vi "GFITS_WriteHeaders_1ext.vi"(0 "ref":u64, 1 "extension":i32, 2 "Database RefNum in":T1, 7 "Keywords":string[][](array[string]), 9 "numer of keywords":i32, 11 "error in (no error)":errorcluster, 12 "expID in":string) -> (6 "ref out":u64, 10 "expID":string, 15 "error out":errorcluster)   [LabVIEW 2016]
uses:
  GFITS_datatypesctl.ctl
  DBSHAND/private/vis/DatabaseHand_RefNum.ctl
  DBSHAND/private/vis/DatabaseHand_Element_Get(bool).vi
panel:
  in  "Types":T2={"TBIT"=1, "TBYTE"=11, "TSTRING"=16, "TSHORT"=21, "TLONG"=41, "TFLOAT"=42, "TDOUBLE"=82, "TCOMPLEX"=83, "TDBLCOMPLEX"=163, "TUINT"=30, "TUSHORT"=20, "TULONG"=40, "TINT"=31, "TSBYTE"=12, "TLONGLONG"=81, "TLOGICAL"=14}
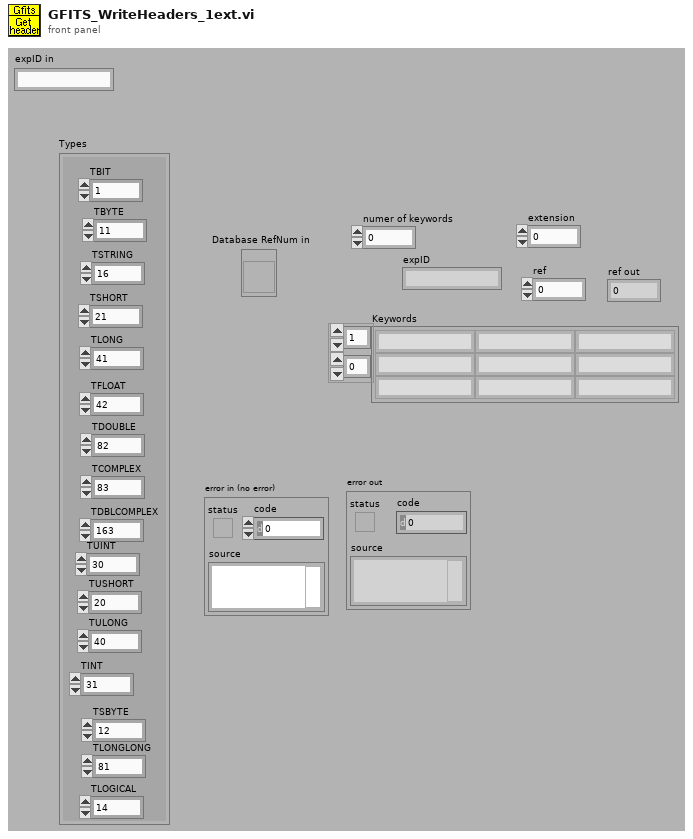
[diagram p1: front panel]
types:
  T1 = typedef "DatabaseHand_RefNum.ctl" = refnum<vi>
  T2 = typedef "GFITS_datatypesctl.ctl" = cluster{"TBIT":i32, "TBYTE":i32, "TSTRING":i32, "TSHORT":i32, "TLONG":i32, "TFLOAT":i32, "TDOUBLE":i32, "TCOMPLEX":i32, "TDBLCOMPLEX":i32, "TUINT":i32, "TUSHORT":i32, "TULONG":i32, "TINT":i32, "TSBYTE":i32, "TLONGLONG":i32, "TLOGICAL":i32}
  T3 = enum16{"clear all", "add extension", "add keyword", "get", "clear extension", "done"}
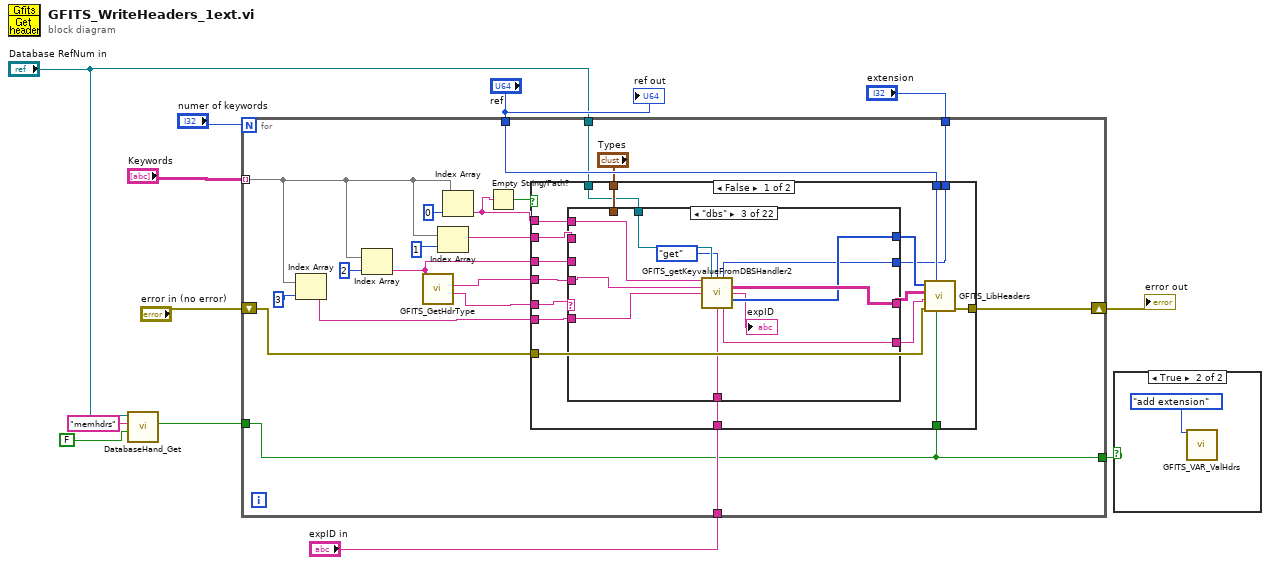
[diagram p0: block diagram]
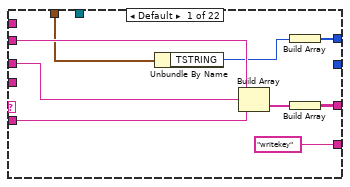
[diagram p3: hidden frame]
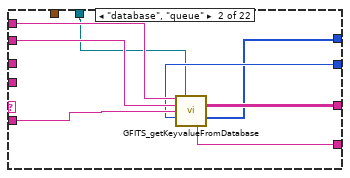
[diagram p4: hidden frame]
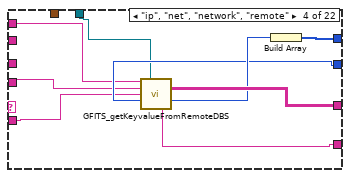
[diagram p5: hidden frame]
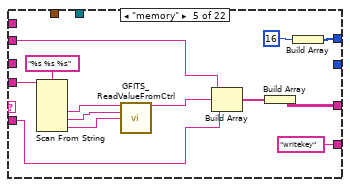
[diagram p6: hidden frame]
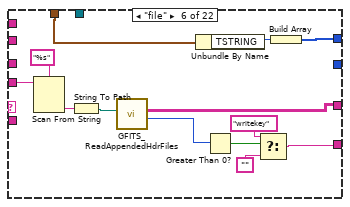
[diagram p7: hidden frame]
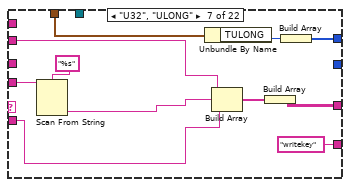
[diagram p8: hidden frame]
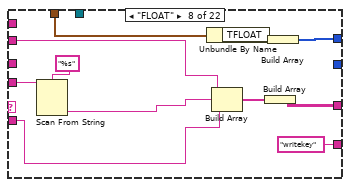
[diagram p9: hidden frame]
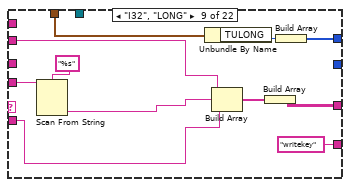
[diagram p10: hidden frame]
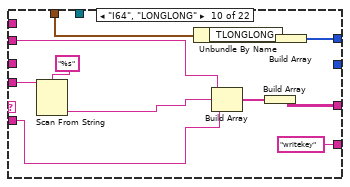
[diagram p11: hidden frame]
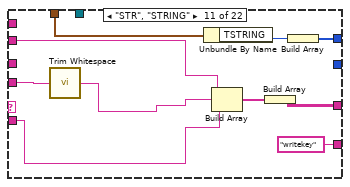
[diagram p12: hidden frame]
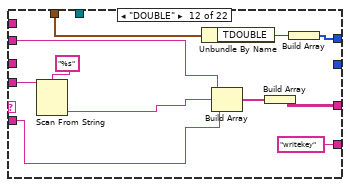
[diagram p13: hidden frame]
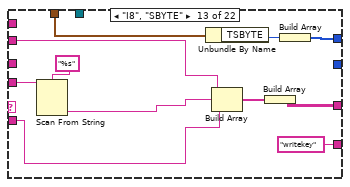
[diagram p14: hidden frame]
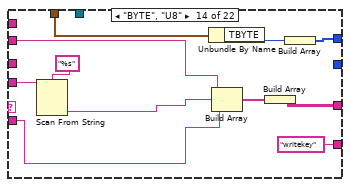
[diagram p15: hidden frame]
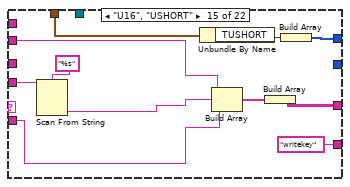
[diagram p16: hidden frame]
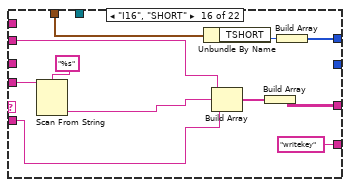
[diagram p17: hidden frame]
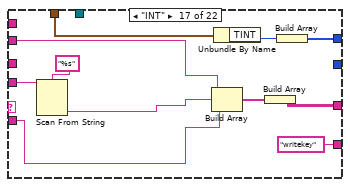
[diagram p18: hidden frame]
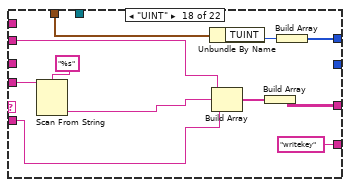
[diagram p19: hidden frame]
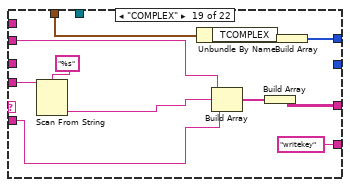
[diagram p20: hidden frame]
diagram:
  n1 = call-poly "DatabaseHand_Get.vi"("default value"=FALSE, "name"="memhdrs", "Database RefNum in"="Database RefNum in") -> ("value"=w2:bool)  [unwired: 2 in, 6 out]
  n2 = for {
    N: "numer of keywords" -> [_]
    tunnel: "Keywords" -> [w26] mode=indexing
    tunnel: "ref" -> [w27]
    tunnel: "extension" -> [w21]
    shift-right: [w16] -> w9
    shift-left: "error in (no error)" -> [w20]
    tunnel: "Database RefNum in" -> [w19]
    tunnel: "expID in" -> [w14]
    tunnel: w2 -> [w13]
    tunnel: [w13] -> w1
    n3 = Index Array(array=w26, index=3 ("Array Index")) -> (element=w28:string)
    n4 = Index Array(array=w26, index=2 ("Array Index")) -> (element=w15:string)
    n5 = call "GFITS_GetHdrType.vi"("keyval"=w15) -> ("type"=w18:string, "keyval out"=w17:string)  [unwired: 9 out]
    n6 = Index Array(array=w26, index=1 ("Array Index")) -> (element=w29:string)
    n7 = Index Array(array=w26, index=0 ("Index")) -> (element=w24:string)
    n8 = Empty String/Path?(string/path=w24) -> (empty?=w23:bool)
    n9 = case shown="False" w23 {
      tunnel: w29 -> [w47 _]
      tunnel: w28 -> [w44 _]
      tunnel: w18 -> [w45 _]
      tunnel: w17 -> [w46 _]
      tunnel: w27 -> [w49 _]
      tunnel: w24 -> [w48 _]
      tunnel: "Types" -> [w41 _]
      tunnel: w21 -> [w35 _]
      tunnel: [w40 w287] -> w16
      tunnel: w20 -> [w39 w287]
      tunnel: w19 -> [w36 _]
      tunnel: w15 -> [w38 _]
      tunnel: w14 -> [w37 _]
      tunnel: w13 -> [w33 _]
      frame False {
        n10 = case shown="\"dbs\"" w45 {
          tunnel: w44 -> [w56 w65 w74 w80 w91 _ w119 w130 w141 w152 w164 w173 w184 w195 w206 w217 w228 w239 w250 w261 w272 w284]
          tunnel: ["writekey" w66 w71 w86 "writekey" ("function to use") w101 "writekey" ("function to use") "writekey" ("function to use") "writekey" ("function to use") "writekey" ("function to use") "writekey" ("function to use") "writekey" ("function to use") "writekey" ("function to use") "writekey" ("function to use") "writekey" ("function to use") "writekey" ("function to use") "writekey" ("function to use") "writekey" ("function to use") "writekey" ("function to use") "writekey" ("function to use") "writekey" ("function to use") "writekey" ("function to use")] -> w42
          tunnel: [w53 w59 w72 w78 w87 w100 w113 w124 w135 w146 w157 w167 w178 w189 w200 w211 w222 w233 w244 w255 w266 w281] -> w43
          tunnel: w47 -> [w57 w62 _ _ w92 _ w120 w131 w142 w153 w165 w174 w185 w196 w207 w218 w229 w240 w251 w262 w273 w285]
          tunnel: w46 -> [_ _ w75 w81 w99 w110 w123 w134 w145 w156 w159 w177 w188 w199 w210 w221 w232 w243 w254 w265 w276 w280]
          tunnel: [w54 w64 w73 w85 w88 w104 w117 w128 w139 w150 w162 w171 w182 w193 w204 w215 w226 w237 w248 w259 w270 w282] -> w34
          tunnel: w48 -> [_ w63 w76 w82 _ _ _ _ _ _ _ _ _ _ _ _ _ _ _ _ _ _]
          tunnel: w41 -> [w52 _ _ _ _ w112 w115 w126 w137 w148 w161 w169 w180 w191 w202 w213 w224 w235 w246 w257 w268 _]
          tunnel: w35 -> [_ w61 w68 w83 _ _ _ _ _ _ _ _ _ _ _ _ _ _ _ _ _ _]
          tunnel: w36 -> [_ w60 w77 w79 _ _ _ _ _ _ _ _ _ _ _ _ _ _ _ _ _ w279]
          tunnel: w38 -> [w50 _ _ _ _ _ _ _ _ _ _ _ _ _ _ _ _ _ _ _ _ _]
          tunnel: w37 -> [_ _ w67 _ _ _ _ _ _ _ _ _ _ _ _ _ _ _ _ _ _ _]
          frame Default {
            n11 = Unbundle By Name(w52) -> ("TSTRING"=w51:i32)
            n12 = Build Array(w57, w50, w56) -> (w55:string[])
            n13 = Build Array(w51) -> (w53:i32[])
            n14 = Build Array(w55) -> (w54:string[][])
          }
          frame "database", "queue" {
            n15 = call "GFITS_getKeyvalueFromDatabase.vi"("key name in header"=w63, "Database RefNum in"=w60, "Keyname"=w62, "comment"=w65, "extension"=w61) -> ("table out"=w64:string[][], "datatype"=w59:u16[], "function to use"=w66:string)  [unwired: 1 in, 7 out]
          }
          frame "dbs" {
            n16 = call "GFITS_getKeyvalueFromDBSHandler2.vi"("key name in header"=w76, "Database RefNum in"=w77, "action"=enum16{"get", "clear"}."get", "extension"=w68, "varname"=w75, "comment"=w74, "expID in"=w67) -> ("table out"=w73:string[][], "expID"=→"expID":string, "datatype"=w72:u16[], "function to use"=w71:string)  [unwired: 3 in, 2 out]
          }
          frame "ip", "net", "network", "remote" {
            n17 = call "GFITS_getKeyvalueFromRemoteDBS.vi"("key name in header"=w82, "Database RefNum in"=w79, "varname"=w81, "comment"=w80, "extension"=w83) -> ("table out"=w85:string[][], "datatype"=w84:u16, "function to use"=w86:string)  [unwired: 1 in, 7 out]
            n18 = Build Array(w84) -> (w78:u16[])
          }
          frame "memory" {
            n19 = Scan From String(format string="%s %s %s" ("Format String"), input string=w99) -> (output 1=w97:string, output 2=w96:string, output 3=w95:string)  [unwired: 2 in, 6 out]
            n20 = call "GFITS_ReadValueFromCtrl.vi"("Vi name"=w97, "Control Name"=w96, "Type"=w95) -> ("Value"=w90:string)  [unwired: 1 in, 11 out]
            n21 = Build Array(w92, w90, w91) -> (w89:string[])
            n22 = Build Array(w89) -> (w88:string[][])
            n23 = Build Array(16 ("datatype")) -> (w87:i32[])
          }
          frame "file" {
            n24 = Scan From String(format string="%s", input string=w110) -> (output 1=w108:string)  [unwired: 2 in, 4 out]
            n25 = String To Path(string=w108) -> (path=w107:path)
            n26 = call "GFITS_ReadAppendedHdrFiles.vi"("Path"=w107) -> ("keywords found"=w106:i32, "Array"=w104:string[][])  [unwired: 1 in, 8 out]
            n27 = Unbundle By Name(w112) -> ("TSTRING"=w111:i32)
            n28 = Greater Than 0?(x=w106) -> (x > 0?=w105:bool)
            n29 = Select(t="writekey" ("function to use"), s=w105, f="") -> (s? t:f=w101:string)
            n30 = Build Array(w111) -> (w100:i32[])
          }
          frame "U32", "ULONG" {
            n31 = Scan From String(format string="%s" ("Format String"), input string=w123) -> (output 1=w116:string)  [unwired: 2 in, 4 out]
            n32 = Unbundle By Name(w115) -> ("TULONG"=w114:i32)
            n33 = Build Array(w120, w116, w119) -> (w118:string[])
            n34 = Build Array(w118) -> (w117:string[][])
            n35 = Build Array(w114) -> (w113:i32[])
          }
          frame "FLOAT" {
            n36 = Scan From String(format string="%s" ("Format String"), input string=w134) -> (output 1=w127:string)  [unwired: 2 in, 4 out]
            n37 = Unbundle By Name(w126) -> ("TFLOAT"=w125:i32)
            n38 = Build Array(w131, w127, w130) -> (w129:string[])
            n39 = Build Array(w129) -> (w128:string[][])
            n40 = Build Array(w125) -> (w124:i32[])
          }
          frame "I32", "LONG" {
            n41 = Scan From String(format string="%s" ("Format String"), input string=w145) -> (output 1=w138:string)  [unwired: 2 in, 4 out]
            n42 = Unbundle By Name(w137) -> ("TULONG"=w136:i32)
            n43 = Build Array(w142, w138, w141) -> (w140:string[])
            n44 = Build Array(w140) -> (w139:string[][])
            n45 = Build Array(w136) -> (w135:i32[])
          }
          frame "I64", "LONGLONG" {
            n46 = Scan From String(format string="%s" ("Format String"), input string=w156) -> (output 1=w149:string)  [unwired: 2 in, 4 out]
            n47 = Unbundle By Name(w148) -> ("TLONGLONG"=w147:i32)
            n48 = Build Array(w153, w149, w152) -> (w151:string[])
            n49 = Build Array(w151) -> (w150:string[][])
            n50 = Build Array(w147) -> (w146:i32[])
          }
          frame "STR", "STRING" {
            n51 = call <vilib>:"Trim Whitespace.vi"("string"=w159) -> ("trimmed string"=w158:string)  [unwired: 1 in]
            n52 = Unbundle By Name(w161) -> ("TSTRING"=w160:i32)
            n53 = Build Array(w165, w158, w164) -> (w163:string[])
            n54 = Build Array(w163) -> (w162:string[][])
            n55 = Build Array(w160) -> (w157:i32[])
          }
          frame "DOUBLE" {
            n56 = Scan From String(format string="%s" ("Format String"), input string=w177) -> (output 1=w170:string)  [unwired: 2 in, 4 out]
            n57 = Unbundle By Name(w169) -> ("TDOUBLE"=w168:i32)
            n58 = Build Array(w174, w170, w173) -> (w172:string[])
            n59 = Build Array(w172) -> (w171:string[][])
            n60 = Build Array(w168) -> (w167:i32[])
          }
          frame "I8", "SBYTE" {
            n61 = Scan From String(format string="%s" ("Format String"), input string=w188) -> (output 1=w181:string)  [unwired: 2 in, 4 out]
            n62 = Unbundle By Name(w180) -> ("TSBYTE"=w179:i32)
            n63 = Build Array(w185, w181, w184) -> (w183:string[])
            n64 = Build Array(w183) -> (w182:string[][])
            n65 = Build Array(w179) -> (w178:i32[])
          }
          frame "BYTE", "U8" {
            n66 = Scan From String(format string="%s" ("Format String"), input string=w199) -> (output 1=w192:string)  [unwired: 2 in, 4 out]
            n67 = Unbundle By Name(w191) -> ("TBYTE"=w190:i32)
            n68 = Build Array(w196, w192, w195) -> (w194:string[])
            n69 = Build Array(w194) -> (w193:string[][])
            n70 = Build Array(w190) -> (w189:i32[])
          }
          frame "U16", "USHORT" {
            n71 = Scan From String(format string="%s" ("Format String"), input string=w210) -> (output 1=w203:string)  [unwired: 2 in, 4 out]
            n72 = Unbundle By Name(w202) -> ("TUSHORT"=w201:i32)
            n73 = Build Array(w207, w203, w206) -> (w205:string[])
            n74 = Build Array(w205) -> (w204:string[][])
            n75 = Build Array(w201) -> (w200:i32[])
          }
          frame "I16", "SHORT" {
            n76 = Scan From String(format string="%s" ("Format String"), input string=w221) -> (output 1=w214:string)  [unwired: 2 in, 4 out]
            n77 = Unbundle By Name(w213) -> ("TSHORT"=w212:i32)
            n78 = Build Array(w218, w214, w217) -> (w216:string[])
            n79 = Build Array(w216) -> (w215:string[][])
            n80 = Build Array(w212) -> (w211:i32[])
          }
          frame "INT" {
            n81 = Scan From String(format string="%s" ("Format String"), input string=w232) -> (output 1=w225:string)  [unwired: 2 in, 4 out]
            n82 = Build Array(w229, w225, w228) -> (w227:string[])
            n83 = Unbundle By Name(w224) -> ("TINT"=w223:i32)
            n84 = Build Array(w227) -> (w226:string[][])
            n85 = Build Array(w223) -> (w222:i32[])
          }
          frame "UINT" {
            n86 = Scan From String(format string="%s" ("Format String"), input string=w243) -> (output 1=w236:string)  [unwired: 2 in, 4 out]
            n87 = Unbundle By Name(w235) -> ("TUINT"=w234:i32)
            n88 = Build Array(w240, w236, w239) -> (w238:string[])
            n89 = Build Array(w238) -> (w237:string[][])
            n90 = Build Array(w234) -> (w233:i32[])
          }
          frame "COMPLEX" {
            n91 = Scan From String(format string="%s" ("Format String"), input string=w254) -> (output 1=w247:string)  [unwired: 2 in, 4 out]
            n92 = Unbundle By Name(w246) -> ("TCOMPLEX"=w245:i32)
            n93 = Build Array(w251, w247, w250) -> (w249:string[])
            n94 = Build Array(w249) -> (w248:string[][])
            n95 = Build Array(w245) -> (w244:i32[])
          }
          frame "DBLCOMPLEX" {
            n96 = Scan From String(format string="%s" ("Format String"), input string=w265) -> (output 1=w258:string)  [unwired: 2 in, 4 out]
            n97 = Unbundle By Name(w257) -> ("TDBLCOMPLEX"=w256:i32)
            n98 = Build Array(w262, w258, w261) -> (w260:string[])
            n99 = Build Array(w260) -> (w259:string[][])
            n100 = Build Array(w256) -> (w255:i32[])
          }
          frame "BIT", "BOOL" {
            n101 = Scan From String(format string="%s" ("Format String"), input string=w276) -> (output 1=w269:string)  [unwired: 2 in, 4 out]
            n102 = Build Array(w273, w269, w272) -> (w271:string[])
            n103 = Unbundle By Name(w268) -> ("TBIT"=w267:i32)
            n104 = Build Array(w271) -> (w270:string[][])
            n105 = Build Array(w267) -> (w266:i32[])
          }
          frame "evaluate", "expression", "operate" {
            n106 = call "GFITS_header_operate.vi"("expression"=w280, "Database RefNum in"=w279) -> ("value"=w277:string, "numeric data type"=w278:i32)  [unwired: 8 out]
            n107 = Build Array(w285, w277, w284) -> (w283:string[])
            n108 = Build Array(w283) -> (w282:string[][])
            n109 = Build Array(w278) -> (w281:i32[])
          }
        }
        n110 = call "GFITS_LibHeaders.vi"("memheaders"=w33, "file ref"=w49, "error in (no error)"=w39, "funtion name"=w42, "Table In"=w34, "data type"=w43) -> ("error out"=w40:errorcluster)  [unwired: 5 out]
      }
      frame True {
      }
    }
  }
  "error out" <- w9
  n111 = case shown="True" w1 {
    frame False {
    }
    frame True {
      n112 = call "GFITS_VAR_ValHdrs.vi"("action"=T3."add extension") -> ()  [unwired: 4 in, 11 out]
    }
  }
  "ref out" <- "ref"
